vi "Write Motor.vi"(8 "error in (no error)":errorcluster, 10 "Motor":T1, 11 "MCB Instrument in":refnum<class "MCB Instrument.lvclass">) -> (0 "error out":errorcluster, 3 "MCB Instrument out":refnum<class "MCB Instrument.lvclass">)   [LabVIEW 2015, in "MCB Instrument.lvlib" / "MCB Instrument.lvclass"]
uses:
  MCB Instrument.lvclass
  Libraries/RDS Child Messages/MCB/MCB Channel.ctl
  MCB Instrument.lvclass/MCB Instrument.ctl
  Libraries/RDS Child Messages/RDS Child Messages.lvlib
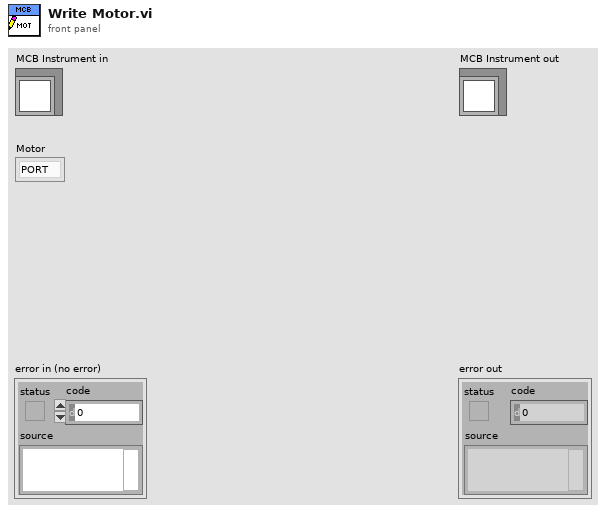
[diagram p1: front panel]
types:
  T1 = typedef "RDS Child Messages.lvlib/MCB Channel.ctl" = enum16{"PORT", "STBD"}
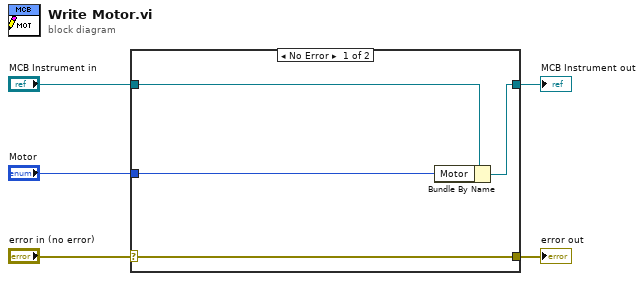
[diagram p0: block diagram]
diagram:
  n1 = case shown="No Error" "error in (no error)" {
    selector: "error in (no error)" -> [w9 w10]
    tunnel: [w9 w10] -> w4
    tunnel: [w7 w11] -> w2
    tunnel: "MCB Instrument in" -> [w8 w11]
    tunnel: "Motor" -> [w6 _]
    frame No Error {
      n2 = Bundle By Name(cluster=w8, "Motor"=w6) -> (w7:refnum<class "MCB Instrument.lvclass">)
    }
    frame Error {
    }
  }
  "error out" <- w4
  "MCB Instrument out" <- w2
